vi "Data_saving.vi"(4 "Boolean":bool, 5 "Sampling Rate":dbl, 6 "File Name":string, 7 "Voltage Sensitivity\n1000 will be 1000":dbl, 9 "Number of Samples Per Channel":i32, 10 "File Path":path, 11 "File name source":path) -> ()   [LabVIEW 2018]
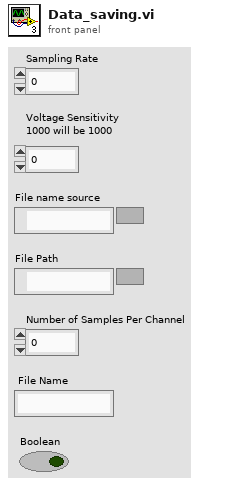
[diagram p1: front panel]
types:
  T1 = enum16{"open", "replace", "create", "open or create", "replace or create", "replace or create with confirmation"}
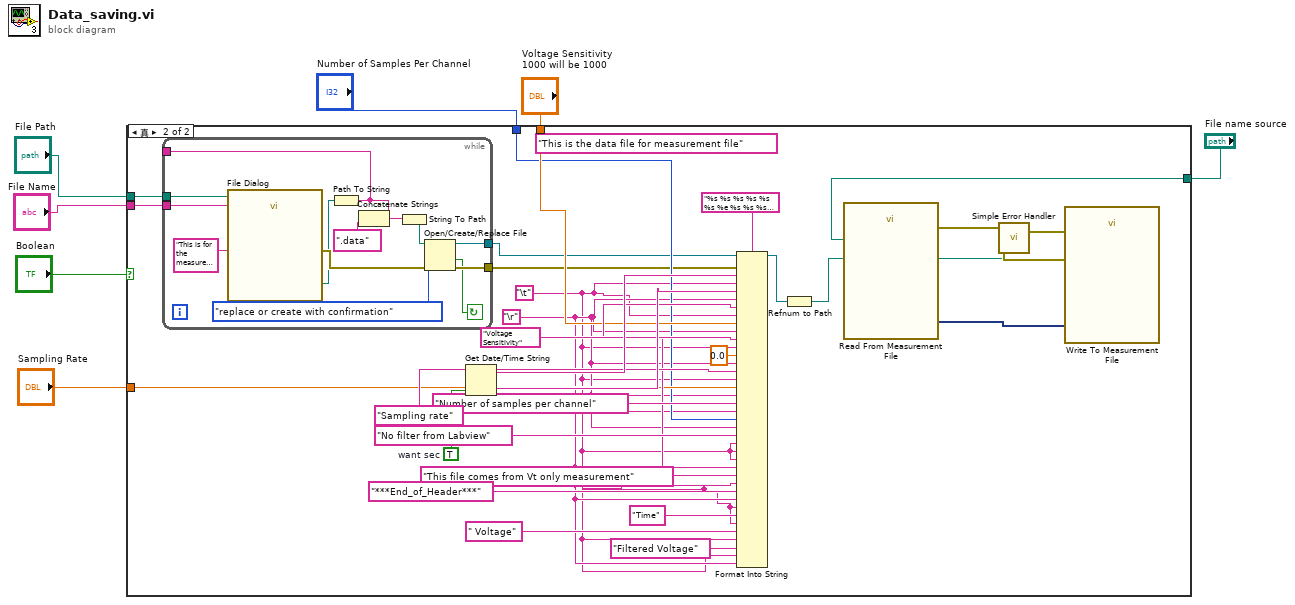
[diagram p0: block diagram]
diagram:
  n1 = case shown="真" "Boolean" {
    tunnel: "File name source" -> [_ w36]
    tunnel: "Voltage Sensitivity\n1000 will be 1000" -> [_ w20]
    tunnel: "Sampling Rate" -> [_ w19]
    tunnel: "Number of Samples Per Channel" -> [_ w15]
    tunnel: "File Name" -> [_ w9]
    tunnel: "File Path" -> [_ w8]
    frame False {
    }
    frame True {
      w13 = "\r"
      w12 = "\t"
      w32 = TRUE  # want sec
      (unwired) "This is the data file for measurement file" ("prompt")
      n2 = while {
        tunnel: [w48] -> w11
        tunnel: [w47] -> w10
        tunnel: [w39] -> _
        tunnel: w9 -> [w38]
        tunnel: w8 -> [w37]
        stop <- w44 continue-if-true
        n3 = call "File Dialog"("start path"=w37, "prompt"="This is for the measurement file", "default name"=w38) -> ("selected path"=w41:path, "error out"=w45:errorcluster)  [unwired: 4 in, 7 out]
        n4 = Path To String(path=w41) -> (string=w39:string)
        n5 = Concatenate Strings(w39, ".data" ("Default File Name 2")) -> (w42:string)
        n6 = String To Path(string=w42) -> (path=w40:path)
        n7 = Open/Create/Replace File(file path (use dialog)=w40, error in=w45, operation (0:open)=T1."replace or create with confirmation") -> (refnum out=w48:refnum<file>, cancelled=w44:bool, error out=w47:errorcluster)  [unwired: 3 out]
      }
      n8 = Get Date/Time String(want seconds? (F)=w32) -> (date string=w31:string, time string=w30:string)  [unwired: 2 out]
      n9 = Format Into String(format string="%s %s %s %s %s %s %e %s %s %s %e %s %s %s %d %s %s %s %d %s %s %s %s %s %s %s %s %s %s %s %s %s %s %s %s %s %s", initial string=w11, error in=w10, w31, w12, w30, w13, "This file comes from Vt only measurement", w12, w20, w13, "Voltage Sensitivity", w12, 0.0 ("input 11"), w13, "Sampling rate", w12, w19, w13, "Number of samples per channel", w12, w15, w13, "No filter from Labview", w12, w12, w12, w13, w12, w13, "***End_of_Header***", w13, w12, "Time", w12, " Voltage", w12, "Filtered Voltage", w12, w13) -> (resulting string=w22:refnum<file>)  [unwired: 1 out]
      n10 = Refnum to Path(1:w22) -> (0:w14:path)
      n11 = call "Read From Measurement File"("Filename"=w36) -> ("error out"=w34:errorcluster, "Signals"=w35:dynamicdata)  [unwired: 5 in, 4 out]
      n12 = call "Write To Measurement File"("File Name"=w14, "error in (no error)"=w34, "Signals"=w35) -> ("error out"=w33:errorcluster)  [unwired: 3 in, 5 out]
      n13 = call <vilib>:"Simple Error Handler.vi"("error in (no error)"=w33) -> ()  [unwired: 1 in, 8 out]
    }
  }
